vi "writeToXML.vi"(8 "error in (no error)":errorcluster, 10 "ClassLabel":string, 11 "Difftrack in":refnum<class "Difftrack.lvclass">) -> (0 "error out":errorcluster, 2 "XML out":string, 3 "Difftrack out":refnum<class "Difftrack.lvclass">)   [LabVIEW 2022 SP3, in "TCSDataDefinitions.lvlib" / "TCSCommand.lvlib" / "TargetConfiguration.lvlib" / "Target.lvlib" / "Difftrack.lvclass"]
uses:
  Difftrack.lvclass
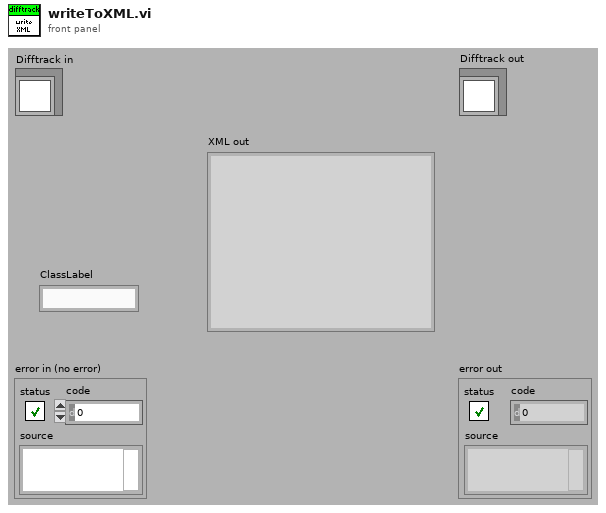
[diagram p1: front panel]
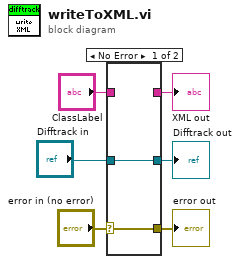
[diagram p0: block diagram]
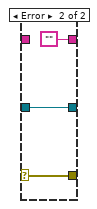
[diagram p2: hidden frame]
diagram:
  n1 = case shown="No Error" "error in (no error)" {
    selector: "error in (no error)" -> [w7 w11]
    tunnel: [w7 w11] -> w5
    tunnel: [w8 w10] -> w4
    tunnel: "Difftrack in" -> [w8 w10]
    tunnel: "ClassLabel" -> [_ _]
    tunnel: [_ ""] -> w2
    frame No Error {
    }
    frame Error {
    }
  }
  "error out" <- w5
  "Difftrack out" <- w4
  "XML out" <- w2
